vi "RT interface_temp.vi"() -> ()   [LabVIEW 2013]
uses:
  <vilib>/Platform/TimedLoop/XDataNode/timing_clust.ctl
  <vilib>/Platform/TimedLoop/XDataNode/nitl_modes.ctl
  <vilib>/Platform/TimedLoop/XDataNode/wakeup.ctl
  <vilib>/rvi/interface/common/niFpgaWaitOnOcc.vi
  <vilib>/FPGAPlugInAG/myRIO-1900/niLvFpga_Open_myRIO-1900.vi
  <vilib>/rvi/interface/common/dynamic/niFpgaDynamicAddResources.vi
  <vilib>/Utility/error.llb/Error Cluster From Error Code.vi
  <vilib>/rvi/errors/niLvFpgaAdjustHostInterfaceError.vi
  <vilib>/FPGAPlugInAG/Dynamic/niLvFpga_Close_Dynamic.vi
  <vilib>/Platform/TimedLoop/XDataNode/XDataNode.xnode
  <vilib>/rvi/interface/nirviOpenFPGA/nirviOpenFPGA.xnode
  FPGA Bitfiles/myRIOAquaponics_FPGATarget_TempmeasDS18B20_8b2VzuBJFnE.lvbitx
  Temp_meas_DS18B20.vi
  <vilib>/rvi/interface/nirviReadWriteControl/nirviReadWriteControl.xnode
  <vilib>/rvi/interface/nirviCloseFPGA/nirviCloseFPGA.xnode
  <vilib>/Platform/TimedLoop/XDataNode/XDNodeRunTimeDep.lvlib
  NiFpgaLv.dll
  <vilib>/rvi/interface/Simulation/niFpgaSimulationCallBeginRW.vi
panel:
  out "Temperature":sgl(graph)
  out "Scratchpad Data":u8[](array[numeric])
  in  "stop":bool
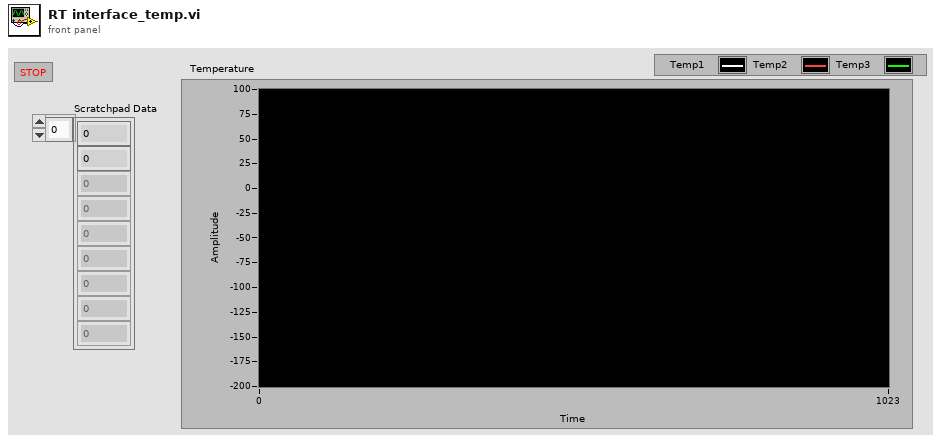
[diagram p1: front panel]
types:
  T1 = typedef "XDNodeRunTimeDep.lvlib/timing_clust.ctl" = cluster{"Expected End [f-1]":u64, "Actual End [f-1]":u64, "Finished Late? [f-1]":bool, "Expected End [i-1]":u64, "Actual End [i-1]":u64, "Finished Late? [i-1]":bool, "Expected Start [i]":u64, "Actual Start [i]":u64, "Expected Start [f]":u64, "Actual Start [f]":u64, "Source Name":string, "Structure Name":string, "Period":i64, "Deadline":i64, "Offset":i64, "Start":i64, "Priority":i32, "Timeout":i32, "Mode":T2, "Wakeup Reason":T3, "Error":errorcluster, "Source Type":string, "Secondary Source Type":string, "Global End Time":u64, "Global Start Time":u64, "Frame Duration":u64, "Iteration Duration":u64, "Assigned CPU":i32, "I/O Scan Engine Mode":u32}
  T2 = typedef "XDNodeRunTimeDep.lvlib/nitl_modes.ctl" = enum32{"No Change", "Process missed periods, maintain original phase", "Discard missed periods, maintain original phase", "Process missed periods, ignore original phase", "Discard missed periods, ignore original phase"}
  T3 = typedef "XDNodeRunTimeDep.lvlib/wakeup.ctl" = enum32{"Normal", "Aborted", "Asynchronous wakeup", "Timing source error", "Timed loop error", "Timeout"}
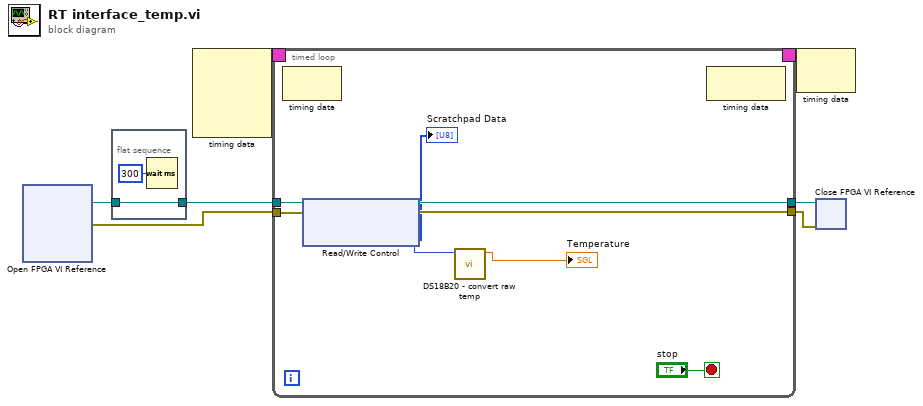
[diagram p0: block diagram]
diagram:
  n1 = xnode "Open FPGA VI Reference"() -> ("FPGA VI Reference Out"=w7:refnum<k20>, "error out"=w1:errorcluster)  [unwired: 2 in]
  n2 = flat-sequence {
    tunnel: w7 -> [w9]
    tunnel: [w9] -> w2
    frame #0 {
      n3 = Wait (ms)(milliseconds to wait=u32 300) -> ()  [unwired: 1 out]
    }
  }
  n4 = node-c288() -> (w6:T1)  [unwired: 4 in]
  n5 = timed-loop {
    tunnel: w2 -> [w16]
    tunnel: w1 -> [w15]
    timing: w6 -> [_]
    timing-out: [_] -> w5
    tunnel: [w14] -> w4
    tunnel: [w13] -> w3
    stop <- "stop" stop-if-true
    n6 = node-c288() -> ()  [unwired: 1 in, 1 out]
    n7 = xnode "Read/Write Control"("FPGA VI Reference In"=w16, "error in"=w15) -> ("FPGA VI Reference Out"=w14:refnum<k20>, "error out"=w13:errorcluster, "Temperature (raw)"=w12:u16, "Scratchpad Data"=→"Scratchpad Data":u8[])
    n8 = call "DS18B20 - convert raw temp.vi"("Raw Temp"=w12) -> ("Temp (C)"=→"Temperature":sgl)  [unwired: 9 in, 1 out]
    n9 = node-c288() -> ()  [unwired: 1 in, 1 out]
  }
  n10 = node-c288(w5) -> ()  [unwired: 1 out]
  n11 = xnode "Close FPGA VI Reference"("FPGA VI Reference In"=w4, "error in"=w3) -> ()  [unwired: 1 out]
